vi "CS++UserContent.vi"   [LabVIEW 2013]
doc: "Place actor and class constants that should be included included in an application on the blockdiagramm."
panel:
  # "Place actor and class constants on the blockdiagramm."
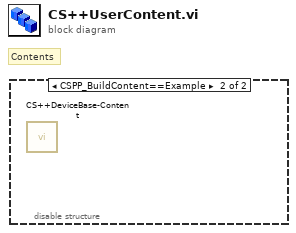
[diagram p0: block diagram]
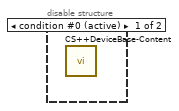
[diagram p2: hidden frame]
diagram:
  # "Contents"
  n1 = disable-structure shown="CSPP_BuildContent==Example" {
    frame condition #0 (active) {
      n2 = call "CS++DeviceBase-Content.vi"() -> ()  [unwired: 12 in]
    }
    frame condition #1 {
      n3 = call "CS++DeviceBase-Content.vi"() -> ()  [unwired: 12 in]
    }
  }
